vi "About.vi"() -> ()   [LabVIEW 2013]
panel:
  out "String":string="Advanced Plotting Toolkit Third-Party License Agreements And Acknowledgements\n========================================================\n\n\"This product includes color specifications and designs developed by\nCynthia Brewer (http://colorbrewer.org/).\"\n\n\nSilk Icons\n----------\n\nThis product makes use of the Silk Icon Set, released by Mark James under the\nCreative Commons Attribution 2.5 License.\n\nhttp://www.famfamfam.com/lab/icons/silk\n\n\nNumPy\n-----\n\nCopyright (c) 2005-2011, NumPy Developers.\nAll rights reserved.\n\nRedistribution and use in source and binary forms, with or without\nmodification, are permitted provided that the following conditions are\nmet:\n\n   Redistributions of source code must retain the above copyright\n       notice, this list of conditions and the following disclaimer.\n\n   Redistributions in binary form must reproduce the above\n       copyright notice, this list of conditions and the following\n       disclaimer in the documentation and/or other materials provided\n       with the distribution.\n\n   Neither the name of the NumPy Developers nor the names of any\n       contributors may be used to endorse or promote products derived\n       from this software without specific prior written permission.\n\nTHIS SOFTWARE IS PROVIDED BY THE COPYRIGHT HOLDERS AND CONTRIBUTORS\n\"AS IS\" AND ANY EXPRESS OR IMPLIED WARRANTIES, INCLUDING, BUT NOT\nLIMITED TO, THE IMPLIED WARRANTIES OF MERCHANTABILITY AND FITNESS FOR\nA PARTICULAR PURPOSE ARE DISCLAIMED. IN NO EVENT SHALL THE COPYRIGHT\nOWNER OR CONTRIBUTORS BE LIABLE FOR ANY DIRECT, INDIRECT, INCIDENTAL,\nSPECIAL, EXEMPLARY, OR CONSEQUENTIAL DAMAGES (INCLUDING, BUT NOT\nLIMITED TO, PROCUREMENT OF SUBSTITUTE GOODS OR SERVICES; LOSS OF USE,\nDATA, OR PROFITS; OR BUSINESS INTERRUPTION) HOWEVER CAUSED AND ON ANY\nTHEORY OF LIABILITY, WHETHER IN CONTRACT, STRICT LIABILITY, OR TORT\n(INCLUDING NEGLIGENCE OR OTHERWISE) ARISING IN ANY WAY OUT OF THE USE\nOF THIS SOFTWARE, EVEN IF ADVISED OF THE POSSIBILITY OF SUCH DAMAGE.\n\n\nNumPy (SafeEval)\n----------------\n\nCopyright 2006 Michael Spencer.  Released under the Python Software\nFoundation License (see \"Python 2.7\", below).\n\n\nNumPy (RandomKit)\n-----------------\n\nCopyright (c) 2003-2005, Jean-Sebastien Roy (js@jeannot.org)\n\nPermission is hereby granted, free of charge, to any person obtaining a\ncopy of this software and associated documentation files (the\n\"Software\"), to deal in the Software without restriction, including\nwithout limitation the rights to use, copy, modify, merge, publish,\ndistribute, sublicense, and/or sell copies of the Software, and to\npermit persons to whom the Software is furnished to do so, subject to\nthe following conditions:\n\nThe above copyright notice and this permission notice shall be included\nin all copies or substantial portions of the Software.\n\nTHE SOFTWARE IS PROVIDED \"AS IS\", WITHOUT WARRANTY OF ANY KIND, EXPRESS\nOR IMPLIED, INCLUDING BUT NOT LIMITED TO THE WARRANTIES OF\nMERCHANTABILITY, FITNESS FOR A PARTICULAR PURPOSE AND NONINFRINGEMENT.\nIN NO EVENT SHALL THE AUTHORS OR COPYRIGHT HOLDERS BE LIABLE FOR ANY\nCLAIM, DAMAGES OR OTHER LIABILITY, WHETHER IN AN ACTION OF CONTRACT,\nTORT OR OTHERWISE, ARISING FROM, OUT OF OR IN CONNECTION WITH THE\nSOFTWARE OR THE USE OR OTHER DEALINGS IN THE SOFTWARE.\n\n\nNumPy (rk_random, rk_seet, Mersenne Twister RNG)\n------------------------------------------------\n\nThe rk_random and rk_seed functions algorithms and the original design of\nthe Mersenne Twister RNG:\n\n  Copyright (C) 1997 - 2002, Makoto Matsumoto and Takuji Nishimura,\n  All rights reserved.\n\n  Redistribution and use in source and binary forms, with or without\n  modification, are permitted provided that the following conditions\n  are met:\n\n  1. Redistributions of source code must retain the above copyright\n  notice, this list of conditions and the following disclaimer.\n\n  2. Redistributions in binary form must reproduce the above copyright\n  notice, this list of conditions and the following disclaimer in the\n  documentation and/or other materials provided with the distribution.\n\n  3. The names of its contributors may not be used to endorse or promote\n  products derived from this software without specific prior written\n  permission.\n\n  THIS SOFTWARE IS PROVIDED BY THE COPYRIGHT HOLDERS AND CONTRIBUTORS\n  \"AS IS\" AND ANY EXPRESS OR IMPLIED WARRANTIES, INCLUDING, BUT NOT\n  LIMITED TO, THE IMPLIED WARRANTIES OF MERCHANTABILITY AND FITNESS FOR\n  A PARTICULAR PURPOSE ARE DISCLAIMED.  IN NO EVENT SHALL THE COPYRIGHT OWNER\n  OR CONTRIBUTORS BE LIABLE FOR ANY DIRECT, INDIRECT, INCIDENTAL, SPECIAL,\n  EXEMPLARY, OR CONSEQUENTIAL DAMAGES (INCLUDING, BUT NOT LIMITED TO,\n  PROCUREMENT OF SUBSTITUTE GOODS OR SERVICES; LOSS OF USE, DATA, OR\n  PROFITS; OR BUSINESS INTERRUPTION) HOWEVER CAUSED AND ON ANY THEORY OF\n  LIABILITY, WHETHER IN CONTRACT, STRICT LIABILITY, OR TORT (INCLUDING\n  NEGLIGENCE OR OTHERWISE) ARISING IN ANY WAY OUT OF THE USE OF THIS\n  SOFTWARE, EVEN IF ADVISED OF THE POSSIBILITY OF SUCH DAMAGE.\n  \n  \nNumPy (MSUN/npy_math)\n---------------------\n\nCopyright (C) 1993 by Sun Microsystems, Inc. All rights reserved.\n\nDeveloped at SunPro, a Sun Microsystems, Inc. business.\nPermission to use, copy, modify, and distribute this\nsoftware is freely granted, provided that this notice\nis preserved.\n\n\nNumPy (npy_math_complex)\n------------------------\n\nCopyright (c) 2007 David Schultz <das@FreeBSD.ORG>\nAll rights reserved.\n\nRedistribution and use in source and binary forms, with or without\nmodification, are permitted provided that the following conditions\nare met:\n1. Redistributions of source code must retain the above copyright\n   notice, this list of conditions and the following disclaimer.\n2. Redistributions in binary form must reproduce the above copyright\n   notice, this list of conditions and the following disclaimer in the\n   documentation and/or other materials provided with the distribution.\n\nTHIS SOFTWARE IS PROVIDED BY THE AUTHOR AND CONTRIBUTORS ``AS IS'' AND\nANY EXPRESS OR IMPLIED WARRANTIES, INCLUDING, BUT NOT LIMITED TO, THE\nIMPLIED WARRANTIES OF MERCHANTABILITY AND FITNESS FOR A PARTICULAR PURPOSE\nARE DISCLAIMED.  IN NO EVENT SHALL THE AUTHOR OR CONTRIBUTORS BE LIABLE\nFOR ANY DIRECT, INDIRECT, INCIDENTAL, SPECIAL, EXEMPLARY, OR CONSEQUENTIAL\nDAMAGES (INCLUDING, BUT NOT LIMITED TO, PROCUREMENT OF SUBSTITUTE GOODS\nOR SERVICES; LOSS OF USE, DATA, OR PROFITS; OR BUSINESS INTERRUPTION)\nHOWEVER CAUSED AND ON ANY THEORY OF LIABILITY, WHETHER IN CONTRACT, STRICT\nLIABILITY, OR TORT (INCLUDING NEGLIGENCE OR OTHERWISE) ARISING IN ANY WAY\nOUT OF THE USE OF THIS SOFTWARE, EVEN IF ADVISED OF THE POSSIBILITY OF\nSUCH DAMAGE.\n\n\nNumPy (mtrand)\n--------------\n\nCopyright 2005 Robert Kern (robert.kern@gmail.com)\n\nPermission is hereby granted, free of charge, to any person obtaining a\ncopy of this software and associated documentation files (the\n\"Software\"), to deal in the Software without restriction, including\nwithout limitation the rights to use, copy, modify, merge, publish,\ndistribute, sublicense, and/or sell copies of the Software, and to\npermit persons to whom the Software is furnished to do so, subject to\nthe following conditions:\n\nThe above copyright notice and this permission notice shall be included\nin all copies or substantial portions of the Software.\n\nTHE SOFTWARE IS PROVIDED \"AS IS\", WITHOUT WARRANTY OF ANY KIND, EXPRESS\nOR IMPLIED, INCLUDING BUT NOT LIMITED TO THE WARRANTIES OF\nMERCHANTABILITY, FITNESS FOR A PARTICULAR PURPOSE AND NONINFRINGEMENT.\nIN NO EVENT SHALL THE AUTHORS OR COPYRIGHT HOLDERS BE LIABLE FOR ANY\nCLAIM, DAMAGES OR OTHER LIABILITY, WHETHER IN AN ACTION OF CONTRACT,\nTORT OR OTHERWISE, ARISING FROM, OUT OF OR IN CONNECTION WITH THE\nSOFTWARE OR THE USE OR OTHER DEALINGS IN THE SOFTWARE.\n\n\nNumPy (fenv)\n------------\n\nCopyright (c) 2004 David Schultz <das@FreeBSD.ORG>\nAll rights reserved.\n\nRedistribution and use in source and binary forms, with or without\nmodification, are permitted provided that the following conditions\nare met:\n1. Redistributions of source code must retain the above copyright\n   notice, this list of conditions and the following disclaimer.\n2. Redistributions in binary form must reproduce the above copyright\n   notice, this list of conditions and the following disclaimer in the\n   documentation and/or other materials provided with the distribution.\n\nTHIS SOFTWARE IS PROVIDED BY THE AUTHOR AND CONTRIBUTORS ``AS IS'' AND\nANY EXPRESS OR IMPLIED WARRANTIES, INCLUDING, BUT NOT LIMITED TO, THE\nIMPLIED WARRANTIES OF MERCHANTABILITY AND FITNESS FOR A PARTICULAR PURPOSE\nARE DISCLAIMED.  IN NO EVENT SHALL THE AUTHOR OR CONTRIBUTORS BE LIABLE\nFOR ANY DIRECT, INDIRECT, INCIDENTAL, SPECIAL, EXEMPLARY, OR CONSEQUENTIAL\nDAMAGES (INCLUDING, BUT NOT LIMITED TO, PROCUREMENT OF SUBSTITUTE GOODS\nOR SERVICES; LOSS OF USE, DATA, OR PROFITS; OR BUSINESS INTERRUPTION)\nHOWEVER CAUSED AND ON ANY THEORY OF LIABILITY, WHETHER IN CONTRACT, STRICT\nLIABILITY, OR TORT (INCLUDING NEGLIGENCE OR OTHERWISE) ARISING IN ANY WAY\nOUT OF THE USE OF THIS SOFTWARE, EVEN IF ADVISED OF THE POSSIBILITY OF\nSUCH DAMAGE.\n\n\nMatplotlib\n----------\n\nLicense agreement for matplotlib 1.3.1 \n\n1. This LICENSE AGREEMENT is between the Matplotlib Development Team\n(“MDT”), and the Individual or Organization (“Licensee”) accessing and\notherwise using matplotlib software in source or binary form and its\nassociated documentation.\n\n2. Subject to the terms and conditions of this License Agreement, MDT\nhereby grants Licensee a nonexclusive, royalty-free, world-wide license\nto reproduce, analyze, test, perform and/or display publicly, prepare\nderivative works, distribute, and otherwise use matplotlib 1.3.1 alone\nor in any derivative version, provided, however, that MDT’s License\nAgreement and MDT’s notice of copyright, i.e., “Copyright (c) 2012-2013\nMatplotlib Development Team; All Rights Reserved” are retained in\nmatplotlib 1.3.1 alone or in any derivative version prepared by\nLicensee.\n\n3. In the event Licensee prepares a derivative work that is based on or\nincorporates matplotlib 1.3.1 or any part thereof, and wants to make the\nderivative work available to others as provided herein, then Licensee\nhereby agrees to include in any such work a brief summary of the changes\nmade to matplotlib 1.3.1.\n\n4. MDT is making matplotlib 1.3.1 available to Licensee on an “AS IS”\nbasis. MDT MAKES NO REPRESENTATIONS OR WARRANTIES, EXPRESS OR IMPLIED.\nBY WAY OF EXAMPLE, BUT NOT LIMITATION, MDT MAKES NO AND DISCLAIMS ANY\nREPRESENTATION OR WARRANTY OF MERCHANTABILITY OR FITNESS FOR ANY\nPARTICULAR PURPOSE OR THAT THE USE OF MATPLOTLIB 1.3.1 WILL NOT INFRINGE\nANY THIRD PARTY RIGHTS.\n\n5. MDT SHALL NOT BE LIABLE TO LICENSEE OR ANY OTHER USERS OF MATPLOTLIB\n1.3.1 FOR ANY INCIDENTAL, SPECIAL, OR CONSEQUENTIAL DAMAGES OR LOSS AS A\nRESULT OF MODIFYING, DISTRIBUTING, OR OTHERWISE USING MATPLOTLIB 1.3.1,\nOR ANY DERIVATIVE THEREOF, EVEN IF ADVISED OF THE POSSIBILITY THEREOF.\n\n6. This License Agreement will automatically terminate upon a material\nbreach of its terms and conditions.\n\n7. Nothing in this License Agreement shall be deemed to create any\nrelationship of agency, partnership, or joint venture between MDT and\nLicensee. This License Agreement does not grant permission to use MDT\ntrademarks or trade name in a trademark sense to endorse or promote\nproducts or services of Licensee, or any third party.\n\n8. By copying, installing or otherwise using matplotlib 1.3.1, Licensee\nagrees to be bound by the terms and conditions of this License Agreement.\n\n\nMatplotlib (PyCXX)\n------------------\n\nCopyright (c) 1998 - 2007, The Regents of the University of California\nProduced at the Lawrence Livermore National Laboratory\nAll rights reserved.\n\nThis file is part of PyCXX. For details,see http:cxx.sourceforge.net/. The\nfull copyright notice is contained in the file COPYRIGHT located at the root\nof the PyCXX distribution.\n\nRedistribution  and  use  in  source  and  binary  forms,  with  or  without\nmodification, are permitted provided that the following conditions are met:\n\n - Redistributions of  source code must  retain the above  copyright notice,\n   this list of conditions and the disclaimer below.\n - Redistributions in binary form must reproduce the above copyright notice,\n   this  list of  conditions  and  the  disclaimer (as noted below)  in  the\n   documentation and/or materials provided with the distribution.\n - Neither the name of the UC/LLNL nor  the names of its contributors may be\n   used to  endorse or  promote products derived from  this software without\n   specific prior written permission.\n\nTHIS SOFTWARE IS PROVIDED BY THE COPYRIGHT  HOLDERS AND CONTRIBUTORS \"AS IS\"\nAND ANY EXPRESS OR  IMPLIED WARRANTIES, INCLUDING,  BUT NOT  LIMITED TO, THE\nIMPLIED WARRANTIES OF MERCHANTABILITY AND  FITNESS FOR A PARTICULAR  PURPOSE\nARE  DISCLAIMED.  IN  NO  EVENT  SHALL  THE  REGENTS  OF  THE  UNIVERSITY OF\nCALIFORNIA, THE U.S.  DEPARTMENT  OF  ENERGY OR CONTRIBUTORS BE  LIABLE  FOR\nANY  DIRECT,  INDIRECT,  INCIDENTAL,  SPECIAL,  EXEMPLARY,  OR CONSEQUENTIAL\nDAMAGES (INCLUDING, BUT NOT  LIMITED TO, PROCUREMENT OF  SUBSTITUTE GOODS OR\nSERVICES; LOSS OF  USE, DATA, OR PROFITS; OR  BUSINESS INTERRUPTION) HOWEVER\nCAUSED  AND  ON  ANY  THEORY  OF  LIABILITY,  WHETHER  IN  CONTRACT,  STRICT\nLIABILITY, OR TORT  (INCLUDING NEGLIGENCE OR OTHERWISE)  ARISING IN ANY  WAY\nOUT OF THE  USE OF THIS SOFTWARE, EVEN IF ADVISED OF THE POSSIBILITY OF SUCH\nDAMAGE.\n\n\nMatplotlib (Agg)\n----------------\n\nThe Anti-Grain Geometry Project\nA high quality rendering engine for C++\nhttp://antigrain.com\n\nAnti-Grain Geometry - Version 2.4 \nCopyright (C) 2002-2005 Maxim Shemanarev (McSeem) \n\nPermission to copy, use, modify, sell and distribute this software \nis granted provided this copyright notice appears in all copies. \nThis software is provided \"as is\" without express or implied\nwarranty, and with no claim as to its suitability for any purpose.\n\n\nMatplotlib (VoronoiDiagram)\n---------------------------\n\nThe author of this software is Steven Fortune.  Copyright (c) 1994 by AT&T\nBell Laboratories.\n\nPermission to use, copy, modify, and distribute this software for any\npurpose without fee is hereby granted, provided that this entire notice\nis included in all copies of any software which is or includes a copy\nor modification of this software and in all copies of the supporting\ndocumentation for such software.\n\nTHIS SOFTWARE IS BEING PROVIDED \"AS IS\", WITHOUT ANY EXPRESS OR IMPLIED\nWARRANTY.  IN PARTICULAR, NEITHER THE AUTHORS NOR AT&T MAKE ANY\nREPRESENTATION OR WARRANTY OF ANY KIND CONCERNING THE MERCHANTABILITY\nOF THIS SOFTWARE OR ITS FITNESS FOR ANY PARTICULAR PURPOSE.\n\n\nMatplotlib (Delauney Triangulation)\n-----------------------------------\n\n(c) Robert Kern, under the SciPy License (follows)\n\nCopyright (c) 2001, 2002 Enthought, Inc.\nAll rights reserved.\n\nCopyright (c) 2003-2013 SciPy Developers.\n\nRedistribution and use in source and binary forms, with or without\nmodification, are permitted provided that the following conditions are\nmet:\n\nRedistributions of source code must retain the above copyright notice,\nthis list of conditions and the following disclaimer. Redistributions in\nbinary form must reproduce the above copyright notice, this list of\nconditions and the following disclaimer in the documentation and/or\nother materials provided with the distribution. Neither the name of\nEnthought nor the names of the SciPy Developers may be used to endorse\nor promote products derived from this software without specific prior\nwritten permission. \n\nTHIS SOFTWARE IS PROVIDED BY THE COPYRIGHT HOLDERS\nAND CONTRIBUTORS “AS IS” AND ANY EXPRESS OR IMPLIED WARRANTIES,\nINCLUDING, BUT NOT LIMITED TO, THE IMPLIED WARRANTIES OF MERCHANTABILITY\nAND FITNESS FOR A PARTICULAR PURPOSE ARE DISCLAIMED. IN NO EVENT SHALL\nTHE REGENTS OR CONTRIBUTORS BE LIABLE FOR ANY DIRECT, INDIRECT,\nINCIDENTAL, SPECIAL, EXEMPLARY, OR CONSEQUENTIAL DAMAGES (INCLUDING, BUT\nNOT LIMITED TO, PROCUREMENT OF SUBSTITUTE GOODS OR SERVICES; LOSS OF\nUSE, DATA, OR PROFITS; OR BUSINESS INTERRUPTION) HOWEVER CAUSED AND ON\nANY THEORY OF LIABILITY, WHETHER IN CONTRACT, STRICT LIABILITY, OR TORT\n(INCLUDING NEGLIGENCE OR OTHERWISE) ARISING IN ANY WAY OUT OF THE USE OF\nTHIS SOFTWARE, EVEN IF ADVISED OF THE POSSIBILITY OF SUCH DAMAGE.\n\n\nMatplotlib (BaKoMa Fonts)\n-------------------------\n\nBaKoMa Fonts Licence\n\n  This licence covers two font packs (known as BaKoMa Fonts Colelction,\n  which is available at `CTAN:fonts/cm/ps-type1/bakoma/'):\n\n    1) BaKoMa-CM (1.1/12-Nov-94)\n       Computer Modern Fonts in PostScript Type 1 and TrueType font formats.\n\n    2) BaKoMa-AMS (1.2/19-Jan-95)\n       AMS TeX fonts in PostScript Type 1 and TrueType font formats.\n   \n  Copyright (C) 1994, 1995, Basil K. Malyshev. All Rights Reserved.\n\n  Permission to copy and distribute these fonts for any purpose is \n  hereby granted without fee, provided that the above copyright notice, \n  author statement and this permission notice appear in all copies of \n  these fonts and related documentation.\n\n  Permission to modify and distribute modified fonts for any purpose is \n  hereby granted without fee, provided that the copyright notice, \n  author statement, this permission notice and location of original \n  fonts (http://www.ctan.org/tex-archive/fonts/cm/ps-type1/bakoma)\n  appear in all copies of modified fonts and related documentation.\n\n  Permission to use these fonts (embedding into PostScript, PDF, SVG\n  and printing by using any software) is hereby granted without fee. \n  It is not required to provide any notices about using these fonts.\n\n Basil K. Malyshev\n INSTITUTE FOR HIGH ENERGY PHYSICS\n IHEP, OMVT\n Moscow Region\n 142281 PROTVINO\n RUSSIA\n\n E-Mail:\tbakoma@mail.ru\n      or\tmalyshev@mail.ihep.ru\n      \n      \nMatplotlib (ColorBrewer)\n------------------------\n\nApache-Style Software License for ColorBrewer Color Schemes\n\nVersion 1.1\n\nCopyright (c) 2002 Cynthia Brewer, Mark Harrower, and The Pennsylvania \nState University. All rights reserved. Redistribution and use in source \nand binary forms, with or without modification, are permitted provided \nthat the following conditions are met:\n\n1. Redistributions as source code must retain the above copyright notice, \nthis list of conditions and the following disclaimer.\n\n2. The end-user documentation included with the redistribution, if any, \nmust include the following acknowledgment: \"This product includes color \nspecifications and designs developed by Cynthia Brewer \n(http://colorbrewer.org/).\" Alternately, this acknowledgment may appear in \nthe software itself, if and wherever such third-party acknowledgments \nnormally appear.\n\n3. The name \"ColorBrewer\" must not be used to endorse or promote products \nderived from this software without prior written permission. For written \npermission, please contact Cynthia Brewer at cbrewer@psu.edu.\n\n4. Products derived from this software may not be called \"ColorBrewer\", \nnor may \"ColorBrewer\" appear in their name, without prior written \npermission of Cynthia Brewer.\n\nTHIS SOFTWARE IS PROVIDED \"AS IS\" AND ANY EXPRESSED OR IMPLIED WARRANTIES, \nINCLUDING, BUT NOT LIMITED TO, THE IMPLIED WARRANTIES OF MERCHANTABILITY \nAND FITNESS FOR A PARTICULAR PURPOSE ARE DISCLAIMED. IN NO EVENT SHALL \nCYNTHIA BREWER, MARK HARROWER, OR THE PENNSYLVANIA STATE UNIVERSITY BE \nLIABLE FOR ANY DIRECT, INDIRECT, INCIDENTAL, SPECIAL, EXEMPLARY, OR \nCONSEQUENTIAL DAMAGES (INCLUDING, BUT NOT LIMITED TO, PROCUREMENT OF \nSUBSTITUTE GOODS OR SERVICES; LOSS OF USE, DATA, OR PROFITS; OR BUSINESS \nINTERRUPTION) HOWEVER CAUSED AND ON ANY THEORY OF LIABILITY, WHETHER IN \nCONTRACT, STRICT LIABILITY, OR TORT (INCLUDING NEGLIGENCE OR OTHERWISE) \nARISING IN ANY WAY OUT OF THE USE OF THIS SOFTWARE, EVEN IF ADVISED OF THE \nPOSSIBILITY OF SUCH DAMAGE.\n\n\nMatplotlib (Enthought Contributions)\n------------------------------------\n\nCopyright (c) 2001, 2002 Enthought, Inc.\n\nAll rights reserved.\n\nRedistribution and use in source and binary forms, with or without\nmodification, are permitted provided that the following conditions are met:\n\n  a. Redistributions of source code must retain the above copyright notice,\n     this list of conditions and the following disclaimer.\n  b. Redistributions in binary form must reproduce the above copyright\n     notice, this list of conditions and the following disclaimer in the\n     documentation and/or other materials provided with the distribution.\n  c. Neither the name of the Enthought nor the names of its contributors\n     may be used to endorse or promote products derived from this software\n     without specific prior written permission.\n\n\nTHIS SOFTWARE IS PROVIDED BY THE COPYRIGHT HOLDERS AND CONTRIBUTORS \"AS IS\"\nAND ANY EXPRESS OR IMPLIED WARRANTIES, INCLUDING, BUT NOT LIMITED TO, THE\nIMPLIED WARRANTIES OF MERCHANTABILITY AND FITNESS FOR A PARTICULAR PURPOSE\nARE DISCLAIMED. IN NO EVENT SHALL THE REGENTS OR CONTRIBUTORS BE LIABLE FOR\nANY DIRECT, INDIRECT, INCIDENTAL, SPECIAL, EXEMPLARY, OR CONSEQUENTIAL\nDAMAGES (INCLUDING, BUT NOT LIMITED TO, PROCUREMENT OF SUBSTITUTE GOODS OR\nSERVICES; LOSS OF USE, DATA, OR PROFITS; OR BUSINESS INTERRUPTION) HOWEVER\nCAUSED AND ON ANY THEORY OF LIABILITY, WHETHER IN CONTRACT, STRICT\nLIABILITY, OR TORT (INCLUDING NEGLIGENCE OR OTHERWISE) ARISING IN ANY WAY\nOUT OF THE USE OF THIS SOFTWARE, EVEN IF ADVISED OF THE POSSIBILITY OF SUCH\nDAMAGE.\n\n\nMatplotlib (Formlayout)\n-----------------------\n\nCopyright (c) 2009 Pierre Raybaut\n\nPermission is hereby granted, free of charge, to any person\nobtaining a copy of this software and associated documentation\nfiles (the \"Software\"), to deal in the Software without\nrestriction, including without limitation the rights to use,\ncopy, modify, merge, publish, distribute, sublicense, and/or sell\ncopies of the Software, and to permit persons to whom the\nSoftware is furnished to do so, subject to the following\nconditions:\n\nThe above copyright notice and this permission notice shall be\nincluded in all copies or substantial portions of the Software.\n\nTHE SOFTWARE IS PROVIDED \"AS IS\", WITHOUT WARRANTY OF ANY KIND,\nEXPRESS OR IMPLIED, INCLUDING BUT NOT LIMITED TO THE WARRANTIES\nOF MERCHANTABILITY, FITNESS FOR A PARTICULAR PURPOSE AND\nNONINFRINGEMENT. IN NO EVENT SHALL THE AUTHORS OR COPYRIGHT\nHOLDERS BE LIABLE FOR ANY CLAIM, DAMAGES OR OTHER LIABILITY,\nWHETHER IN AN ACTION OF CONTRACT, TORT OR OTHERWISE, ARISING\nFROM, OUT OF OR IN CONNECTION WITH THE SOFTWARE OR THE USE OR\nOTHER DEALINGS IN THE SOFTWARE.\n\n\nMatplotlib (STIX Fonts)\n-----------------------\n\nCopyright (c) 2001-2010 by the STI Pub Companies, consisting of the American\nInstitute of Physics, the American Chemical Society, the American Mathematical\nSociety, the American Physical Society, Elsevier, Inc., and The Institute of\nElectrical and Electronic Engineers, Inc. (www.stixfonts.org), with Reserved\nFont Name STIX Fonts, STIX Fonts (TM) is a  trademark of The Institute of\nElectrical and Electronics Engineers, Inc.\n\nPortions copyright (c) 1998-2003 by MicroPress, Inc. (www.micropress-inc.com),\nwith Reserved Font Name TM Math. To obtain additional mathematical fonts, please\ncontact MicroPress, Inc., 68-30 Harrow Street, Forest Hills, NY 11375, USA,\nPhone: (718) 575-1816.\n\nPortions copyright (c) 1990 by Elsevier, Inc.\n\nThis Font Software is licensed under the SIL Open Font License, Version 1.1.\nThis license is copied below, and is also available with a FAQ at:\nhttp://scripts.sil.org/OFL\n\n-----------------------------------------------------------\nSIL OPEN FONT LICENSE Version 1.1 - 26 February 2007\n-----------------------------------------------------------\n\nPREAMBLE\nThe goals of the Open Font License (OFL) are to stimulate worldwide\ndevelopment of collaborative font projects, to support the font creation\nefforts of academic and linguistic communities, and to provide a free and\nopen framework in which fonts may be shared and improved in partnership\nwith others.\n\nThe OFL allows the licensed fonts to be used, studied, modified and\nredistributed freely as long as they are not sold by themselves. The\nfonts, including any derivative works, can be bundled, embedded,\nredistributed and/or sold with any software provided that any reserved\nnames are not used by derivative works. The fonts and derivatives,\nhowever, cannot be released under any other type of license. The\nrequirement for fonts to remain under this license does not apply\nto any document created using the fonts or their derivatives.\n\nDEFINITIONS\n\"Font Software\" refers to the set of files released by the Copyright\nHolder(s) under this license and clearly marked as such. This may\ninclude source files, build scripts and documentation.\n\n\"Reserved Font Name\" refers to any names specified as such after the\ncopyright statement(s).\n\n\"Original Version\" refers to the collection of Font Software components as\ndistributed by the Copyright Holder(s).\n\n\"Modified Version\" refers to any derivative made by adding to, deleting,\nor substituting -- in part or in whole -- any of the components of the\nOriginal Version, by changing formats or by porting the Font Software to a\nnew environment.\n\n\"Author\" refers to any designer, engineer, programmer, technical\nwriter or other person who contributed to the Font Software.\n\nPERMISSION & CONDITIONS\nPermission is hereby granted, free of charge, to any person obtaining\na copy of the Font Software, to use, study, copy, merge, embed, modify,\nredistribute, and sell modified and unmodified copies of the Font\nSoftware, subject to the following conditions:\n\n1) Neither the Font Software nor any of its individual components,\nin Original or Modified Versions, may be sold by itself.\n\n2) Original or Modified Versions of the Font Software may be bundled,\nredistributed and/or sold with any software, provided that each copy\ncontains the above copyright notice and this license. These can be\nincluded either as stand-alone text files, human-readable headers or\nin the appropriate machine-readable metadata fields within text or\nbinary files as long as those fields can be easily viewed by the user.\n\n3) No Modified Version of the Font Software may use the Reserved Font\nName(s) unless explicit written permission is granted by the corresponding\nCopyright Holder. This restriction only applies to the primary font name as\npresented to the users.\n\n4) The name(s) of the Copyright Holder(s) or the Author(s) of the Font\nSoftware shall not be used to promote, endorse or advertise any\nModified Version, except to acknowledge the contribution(s) of the\nCopyright Holder(s) and the Author(s) or with their explicit written\npermission.\n\n5) The Font Software, modified or unmodified, in part or in whole,\nmust be distributed entirely under this license, and must not be\ndistributed under any other license. The requirement for fonts to\nremain under this license does not apply to any document created\nusing the Font Software.\n\nTERMINATION\nThis license becomes null and void if any of the above conditions are\nnot met.\n\nDISCLAIMER\nTHE FONT SOFTWARE IS PROVIDED \"AS IS\", WITHOUT WARRANTY OF ANY KIND,\nEXPRESS OR IMPLIED, INCLUDING BUT NOT LIMITED TO ANY WARRANTIES OF\nMERCHANTABILITY, FITNESS FOR A PARTICULAR PURPOSE AND NONINFRINGEMENT\nOF COPYRIGHT, PATENT, TRADEMARK, OR OTHER RIGHT. IN NO EVENT SHALL THE\nCOPYRIGHT HOLDER BE LIABLE FOR ANY CLAIM, DAMAGES OR OTHER LIABILITY,\nINCLUDING ANY GENERAL, SPECIAL, INDIRECT, INCIDENTAL, OR CONSEQUENTIAL\nDAMAGES, WHETHER IN AN ACTION OF CONTRACT, TORT OR OTHERWISE, ARISING\nFROM, OUT OF THE USE OR INABILITY TO USE THE FONT SOFTWARE OR FROM\nOTHER DEALINGS IN THE FONT SOFTWARE.\n\n\nMatplotlib (GIST/Yorick Colormaps)\n----------------------------------\n\n  Copyright (c) 1996.  The Regents of the University of California.\n\t\t\t All rights reserved.\n\nPermission to use, copy, modify, and distribute this software for any\npurpose without fee is hereby granted, provided that this entire\nnotice is included in all copies of any software which is or includes\na copy or modification of this software and in all copies of the\nsupporting documentation for such software.\n\nThis work was produced at the University of California, Lawrence\nLivermore National Laboratory under contract no. W-7405-ENG-48 between\nthe U.S. Department of Energy and The Regents of the University of\nCalifornia for the operation of UC LLNL.\n\n\n\t\t\t      DISCLAIMER\n\nThis software was prepared as an account of work sponsored by an\nagency of the United States Government.  Neither the United States\nGovernment nor the University of California nor any of their\nemployees, makes any warranty, express or implied, or assumes any\nliability or responsibility for the accuracy, completeness, or\nusefulness of any information, apparatus, product, or process\ndisclosed, or represents that its use would not infringe\nprivately-owned rights.  Reference herein to any specific commercial\nproducts, process, or service by trade name, trademark, manufacturer,\nor otherwise, does not necessarily constitute or imply its\nendorsement, recommendation, or favoring by the United States\nGovernment or the University of California.  The views and opinions of\nauthors expressed herein do not necessarily state or reflect those of\nthe United States Government or the University of California, and\nshall not be used for advertising or product endorsement purposes.\n\n\n\t\t\t\tAUTHOR\n\nDavid H. Munro wrote Yorick and Gist.  Berkeley Yacc (byacc) generated\nthe Yorick parser.  The routines in Math are from LAPACK and FFTPACK;\nMathC contains C translations by David H. Munro.  The algorithms for\nYorick's random number generator and several special functions in\nYorick/include were taken from Numerical Recipes by Press, et. al.,\nalthough the Yorick implementations are unrelated to those in\nNumerical Recipes.  A small amount of code in Gist was adapted from\nthe X11R4 release, copyright M.I.T. -- the complete copyright notice\nmay be found in the (unused) file Gist/host.c.\n\n\nMatplotlib (Pnpoly)\n-------------------\n\nCopyright (c) 1970-2003, Wm. Randolph Franklin\n\nPermission is hereby granted, free of charge, to any person obtaining\na copy of this software and associated documentation files (the\n\"Software\"), to deal in the Software without restriction, including\nwithout limitation the rights to use, copy, modify, merge, publish,\ndistribute, sublicense, and/or sell copies of the Software, and to\npermit persons to whom the Software is furnished to do so, subject to\nthe following conditions:\n\n   1. Redistributions of source code must retain the above copyright\n      notice, this list of conditions and the following disclaimers.\n   2. Redistributions in binary form must reproduce the above\n      copyright notice in the documentation and/or other materials\n      provided with the distribution.\n   3. The name of W. Randolph Franklin may not be used to endorse or\n      promote products derived from this Software without specific\n      prior written permission. \n\nTHE SOFTWARE IS PROVIDED \"AS IS\", WITHOUT WARRANTY OF ANY KIND,\nEXPRESS OR IMPLIED, INCLUDING BUT NOT LIMITED TO THE WARRANTIES OF\nMERCHANTABILITY, FITNESS FOR A PARTICULAR PURPOSE AND\nNONINFRINGEMENT. IN NO EVENT SHALL THE AUTHORS OR COPYRIGHT HOLDERS BE\nLIABLE FOR ANY CLAIM, DAMAGES OR OTHER LIABILITY, WHETHER IN AN ACTION\nOF CONTRACT, TORT OR OTHERWISE, ARISING FROM, OUT OF OR IN CONNECTION\nWITH THE SOFTWARE OR THE USE OR OTHER DEALINGS IN THE SOFTWARE.\n\n\nMatplotlib (ttconv)\n-------------------\n\nCopyright 1995, Trinity College Computing Center.\nWritten by David Chappell.\n\nPermission to use, copy, modify, and distribute this software and its\ndocumentation for any purpose and without fee is hereby granted, provided\nthat the above copyright notice appear in all copies and that both that\ncopyright notice and this permission notice appear in supporting\ndocumentation.  This software is provided \"as is\" without express or\nimplied warranty.\n\n\nMatplotlib (Bitstream Vera)\n---------------------------\n\nBitstream Vera Fonts Copyright\n\nThe fonts have a generous copyright, allowing derivative works (as\nlong as \"Bitstream\" or \"Vera\" are not in the names), and full\nredistribution (so long as they are not sold by themselves). They\ncan be be bundled, redistributed and sold with any software.\n\nThe fonts are distributed under the following copyright:\n\nCopyright (c) 2003 by Bitstream, Inc. All Rights Reserved. Bitstream\nVera is a trademark of Bitstream, Inc.\n\nPermission is hereby granted, free of charge, to any person obtaining\na copy of the fonts accompanying this license (\"Fonts\") and associated\ndocumentation files (the \"Font Software\"), to reproduce and distribute\nthe Font Software, including without limitation the rights to use,\ncopy, merge, publish, distribute, and/or sell copies of the Font\nSoftware, and to permit persons to whom the Font Software is furnished\nto do so, subject to the following conditions:\n\nThe above copyright and trademark notices and this permission notice\nshall be included in all copies of one or more of the Font Software\ntypefaces.\n\nThe Font Software may be modified, altered, or added to, and in\nparticular the designs of glyphs or characters in the Fonts may be\nmodified and additional glyphs or characters may be added to the\nFonts, only if the fonts are renamed to names not containing either\nthe words \"Bitstream\" or the word \"Vera\".\n\nThis License becomes null and void to the extent applicable to Fonts\nor Font Software that has been modified and is distributed under the\n\"Bitstream Vera\" names.\n\nThe Font Software may be sold as part of a larger software package but\nno copy of one or more of the Font Software typefaces may be sold by\nitself.\n\nTHE FONT SOFTWARE IS PROVIDED \"AS IS\", WITHOUT WARRANTY OF ANY KIND,\nEXPRESS OR IMPLIED, INCLUDING BUT NOT LIMITED TO ANY WARRANTIES OF\nMERCHANTABILITY, FITNESS FOR A PARTICULAR PURPOSE AND NONINFRINGEMENT\nOF COPYRIGHT, PATENT, TRADEMARK, OR OTHER RIGHT. IN NO EVENT SHALL\nBITSTREAM OR THE GNOME FOUNDATION BE LIABLE FOR ANY CLAIM, DAMAGES OR\nOTHER LIABILITY, INCLUDING ANY GENERAL, SPECIAL, INDIRECT, INCIDENTAL,\nOR CONSEQUENTIAL DAMAGES, WHETHER IN AN ACTION OF CONTRACT, TORT OR\nOTHERWISE, ARISING FROM, OUT OF THE USE OR INABILITY TO USE THE FONT\nSOFTWARE OR FROM OTHER DEALINGS IN THE FONT SOFTWARE.\n\nExcept as contained in this notice, the names of Gnome, the Gnome\nFoundation, and Bitstream Inc., shall not be used in advertising or\notherwise to promote the sale, use or other dealings in this Font\nSoftware without prior written authorization from the Gnome Foundation\nor Bitstream Inc., respectively. For further information, contact:\nfonts at gnome dot org.\n\n\nMatplotlib (14 PDF Core Fonts)\n------------------------------\n\nFont Metrics for the 14 PDF Core Fonts (README from the Matplotlib\npackage):\n\nThis directory contains font metrics for the 14 PDF Core Fonts,\ndownloaded from Adobe. The title and this paragraph were added by\nMatplotlib developers. The download URL was\n<http://partners.adobe.com/public/developer/font/index.html>.\n\nThis file and the 14 PostScript(R) AFM files it accompanies may be used,\ncopied, and distributed for any purpose and without charge, with or\nwithout modification, provided that all copyright notices are retained;\nthat the AFM files are not distributed without this file; that all\nmodifications to this file or any of the AFM files are prominently noted\nin the modified file(s); and that this paragraph is not modified. Adobe\nSystems has no responsibility or obligation to support the use of the\nAFM files.\n\n\nMatplotlib (IPython Numutils)\n-----------------------------\n\nCopyright (c) 2001-2004, Fernando Perez. <Fernando.Perez@colorado.edu>\nAll rights reserved.\n\nThis license was generated from the BSD license template as found in:\nhttp://www.opensource.org/licenses/bsd-license.php\n\nRedistribution and use in source and binary forms, with or without\nmodification, are permitted provided that the following conditions are met:\n\n    Redistributions of source code must retain the above copyright notice,\n      this list of conditions and the following disclaimer.\n\n    Redistributions in binary form must reproduce the above copyright\n      notice, this list of conditions and the following disclaimer in the\n      documentation and/or other materials provided with the distribution.\n\n    Neither the name of the IPython project nor the names of its\n      contributors may be used to endorse or promote products derived from\n      this software without specific prior written permission.\n\nTHIS SOFTWARE IS PROVIDED BY THE COPYRIGHT HOLDERS AND CONTRIBUTORS \"AS IS\"\nAND ANY EXPRESS OR IMPLIED WARRANTIES, INCLUDING, BUT NOT LIMITED TO, THE\nIMPLIED WARRANTIES OF MERCHANTABILITY AND FITNESS FOR A PARTICULAR PURPOSE ARE\nDISCLAIMED. IN NO EVENT SHALL THE COPYRIGHT OWNER OR CONTRIBUTORS BE LIABLE\nFOR ANY DIRECT, INDIRECT, INCIDENTAL, SPECIAL, EXEMPLARY, OR CONSEQUENTIAL\nDAMAGES (INCLUDING, BUT NOT LIMITED TO, PROCUREMENT OF SUBSTITUTE GOODS OR\nSERVICES; LOSS OF USE, DATA, OR PROFITS; OR BUSINESS INTERRUPTION) HOWEVER\nCAUSED AND ON ANY THEORY OF LIABILITY, WHETHER IN CONTRACT, STRICT LIABILITY,\nOR TORT (INCLUDING NEGLIGENCE OR OTHERWISE) ARISING IN ANY WAY OUT OF THE USE\nOF THIS SOFTWARE, EVEN IF ADVISED OF THE POSSIBILITY OF SUCH DAMAGE.\n\n\nPython 2.7\n----------\n\nPYTHON SOFTWARE FOUNDATION LICENSE VERSION 2\n--------------------------------------------\n\n1. This LICENSE AGREEMENT is between the Python Software Foundation\n(\"PSF\"), and the Individual or Organization (\"Licensee\") accessing and\notherwise using this software (\"Python\") in source or binary form and\nits associated documentation.\n\n2. Subject to the terms and conditions of this License Agreement, PSF\nhereby grants Licensee a nonexclusive, royalty-free, world-wide\nlicense to reproduce, analyze, test, perform and/or display publicly,\nprepare derivative works, distribute, and otherwise use Python\nalone or in any derivative version, provided, however, that PSF's\nLicense Agreement and PSF's notice of copyright, i.e., \"Copyright (c)\n2001, 2002, 2003, 2004, 2005, 2006 Python Software Foundation; All Rights\nReserved\" are retained in Python alone or in any derivative version \nprepared by Licensee.\n\n3. In the event Licensee prepares a derivative work that is based on\nor incorporates Python or any part thereof, and wants to make\nthe derivative work available to others as provided herein, then\nLicensee hereby agrees to include in any such work a brief summary of\nthe changes made to Python.\n\n4. PSF is making Python available to Licensee on an \"AS IS\"\nbasis.  PSF MAKES NO REPRESENTATIONS OR WARRANTIES, EXPRESS OR\nIMPLIED.  BY WAY OF EXAMPLE, BUT NOT LIMITATION, PSF MAKES NO AND\nDISCLAIMS ANY REPRESENTATION OR WARRANTY OF MERCHANTABILITY OR FITNESS\nFOR ANY PARTICULAR PURPOSE OR THAT THE USE OF PYTHON WILL NOT\nINFRINGE ANY THIRD PARTY RIGHTS.\n\n5. PSF SHALL NOT BE LIABLE TO LICENSEE OR ANY OTHER USERS OF PYTHON\nFOR ANY INCIDENTAL, SPECIAL, OR CONSEQUENTIAL DAMAGES OR LOSS AS\nA RESULT OF MODIFYING, DISTRIBUTING, OR OTHERWISE USING PYTHON,\nOR ANY DERIVATIVE THEREOF, EVEN IF ADVISED OF THE POSSIBILITY THEREOF.\n\n6. This License Agreement will automatically terminate upon a material\nbreach of its terms and conditions.\n\n7. Nothing in this License Agreement shall be deemed to create any\nrelationship of agency, partnership, or joint venture between PSF and\nLicensee.  This License Agreement does not grant permission to use PSF\ntrademarks or trade name in a trademark sense to endorse or promote\nproducts or services of Licensee, or any third party.\n\n8. By copying, installing or otherwise using Python, Licensee\nagrees to be bound by the terms and conditions of this License\nAgreement.\n\n\nPyWin32\n-------\n\nCopyright (c) 1996-2008, Greg Stein and Mark Hammond.\nAll rights reserved.\n\nRedistribution and use in source and binary forms, with or without \nmodification, are permitted provided that the following conditions \nare met:\n\nRedistributions of source code must retain the above copyright notice, \nthis list of conditions and the following disclaimer.\n\nRedistributions in binary form must reproduce the above copyright \nnotice, this list of conditions and the following disclaimer in \nthe documentation and/or other materials provided with the distribution.\n\nNeither names of Greg Stein, Mark Hammond nor the name of contributors may be used \nto endorse or promote products derived from this software without \nspecific prior written permission. \n\nTHIS SOFTWARE IS PROVIDED BY THE COPYRIGHT HOLDERS AND CONTRIBUTORS ``AS\nIS'' AND ANY EXPRESS OR IMPLIED WARRANTIES, INCLUDING, BUT NOT LIMITED\nTO, THE IMPLIED WARRANTIES OF MERCHANTABILITY AND FITNESS FOR A\nPARTICULAR PURPOSE ARE DISCLAIMED. IN NO EVENT SHALL THE REGENTS OR\nCONTRIBUTORS BE LIABLE FOR ANY DIRECT, INDIRECT, INCIDENTAL, SPECIAL,\nEXEMPLARY, OR CONSEQUENTIAL DAMAGES (INCLUDING, BUT NOT LIMITED TO,\nPROCUREMENT OF SUBSTITUTE GOODS OR SERVICES; LOSS OF USE, DATA, OR\nPROFITS; OR BUSINESS INTERRUPTION) HOWEVER CAUSED AND ON ANY THEORY OF\nLIABILITY, WHETHER IN CONTRACT, STRICT LIABILITY, OR TORT (INCLUDING\nNEGLIGENCE OR OTHERWISE) ARISING IN ANY WAY OUT OF THE USE OF THIS\nSOFTWARE, EVEN IF ADVISED OF THE POSSIBILITY OF SUCH DAMAGE.\n\n\nPyWin32 (Scintilla portions)\n----------------------------\n\nCopyright 1998-2003 by Neil Hodgson <neilh@scintilla.org>\n\nAll Rights Reserved \n\nPermission to use, copy, modify, and distribute this software and its \ndocumentation for any purpose and without fee is hereby granted, \nprovided that the above copyright notice appear in all copies and that \nboth that copyright notice and this permission notice appear in \nsupporting documentation. \n\nNEIL HODGSON DISCLAIMS ALL WARRANTIES WITH REGARD TO THIS \nSOFTWARE, INCLUDING ALL IMPLIED WARRANTIES OF MERCHANTABILITY \nAND FITNESS, IN NO EVENT SHALL NEIL HODGSON BE LIABLE FOR ANY \nSPECIAL, INDIRECT OR CONSEQUENTIAL DAMAGES OR ANY DAMAGES \nWHATSOEVER RESULTING FROM LOSS OF USE, DATA OR PROFITS, \nWHETHER IN AN ACTION OF CONTRACT, NEGLIGENCE OR OTHER \nTORTIOUS ACTION, ARISING OUT OF OR IN CONNECTION WITH THE USE \nOR PERFORMANCE OF THIS SOFTWARE.\n\n\nPyWin32 (win32wnet)\n-------------------\n\nCopyright (c) 1998-1999 Cisco Systems, Inc. All Rights Reserved\nPermission to use, copy, modify, and distribute this software and its\ndocumentation for any purpose and without fee is hereby granted,\nprovided that the above copyright notice appear in all copies and that\nboth that copyright notice and this permission notice appear in\nsupporting documentation.\n\nCISCO SYSTEMS, INC. DISCLAIMS ALL WARRANTIES WITH REGARD TO THIS\nSOFTWARE, INCLUDING ALL IMPLIED WARRANTIES OF MERCHANTABILITY AND\nFITNESS. IN NO EVENT SHALL CISCO SYSTEMS BE LIABLE FOR ANY LOST REVENUE, \nPROFIT OR DATA, OR FOR SPECIAL, INDIRECT, CONSEQUENTIAL OR INCIDENTAL\nDAMAGES OR ANY OTHER DAMAGES WHATSOEVER, HOWEVER CAUSED AND REGARDLESS\nOF THE THEORY OF LIABILITY, ARISING OUT OF OR IN CONNECTION\nWITH THE USE OR PERFORMANCE OF THIS SOFTWARE.\n\n\nPyWin32 (win32dlgdyn)\n---------------------\n\nCopyright (C) 1995 by Motek Information Systems, Beverly Hills, CA, USA\n\n                      All Rights Reserved\n\nPermission to use, copy, modify, and distribute this software and its \ndocumentation for any purpose and without fee is hereby granted, \nprovided that the above copyright notice and the two paragraphs following\nit appear in all copies, and that the name of Motek Information Systems\nnot be used in advertising or publicity pertaining to distribution of the\nsoftware without specific, written prior permission.\n\nMOTEK INFORMATION SYSTEMS DISCLAIMS ALL WARRANTIES WITH REGARD TO\nTHIS SOFTWARE, INCLUDING ALL IMPLIED WARRANTIES OF MERCHANTABILITY AND\nFITNESS, IN NO EVENT SHALL MOTEK BE LIABLE FOR ANY SPECIAL, INDIRECT OR\nCONSEQUENTIAL DAMAGES OR ANY DAMAGES WHATSOEVER RESULTING FROM LOSS OF USE,\nDATA OR PROFITS, WHETHER IN AN ACTION OF CONTRACT, NEGLIGENCE OR OTHER\nTORTIOUS ACTION, ARISING OUT OF OR IN CONNECTION WITH THE USE OR\nPERFORMANCE OF THIS SOFTWARE.\n\n\nPyWin32 (stdin)\n---------------\n\nCopyright (c) 2000 David Abrahams. Permission to copy, use, modify, sell\nand distribute this software is granted provided this copyright\nnotice appears in all copies. This software is provided \"as is\" without\nexpress or implied warranty, and with no claim as to its suitability for\nany purpose.\n\n\nPillow\n------\n\nThe Python Imaging Library (PIL) is\n\n   Copyright (c) 1997-2011 by Secret Labs AB \n   Copyright (c) 1995-2011 by Fredrik Lundh\n\nBy obtaining, using, and/or copying this software and/or its associated\ndocumentation, you agree that you have read, understood, and will comply\nwith the following terms and conditions:\n\nPermission to use, copy, modify, and distribute this software and its\nassociated documentation for any purpose and without fee is hereby\ngranted, provided that the above copyright notice appears in all copies,\nand that both that copyright notice and this permission notice appear in\nsupporting documentation, and that the name of Secret Labs AB or the\nauthor not be used in advertising or publicity pertaining to\ndistribution of the software without specific, written prior permission.\n\nSECRET LABS AB AND THE AUTHOR DISCLAIMS ALL WARRANTIES WITH REGARD TO\nTHIS SOFTWARE, INCLUDING ALL IMPLIED WARRANTIES OF MERCHANTABILITY AND\nFITNESS. IN NO EVENT SHALL SECRET LABS AB OR THE AUTHOR BE LIABLE FOR\nANY SPECIAL, INDIRECT OR CONSEQUENTIAL DAMAGES OR ANY DAMAGES WHATSOEVER\nRESULTING FROM LOSS OF USE, DATA OR PROFITS, WHETHER IN AN ACTION OF\nCONTRACT, NEGLIGENCE OR OTHER TORTIOUS ACTION, ARISING OUT OF OR IN\nCONNECTION WITH THE USE OR PERFORMANCE OF THIS SOFTWARE.\n\n\nPillow (QuantOctree)\n--------------------\n\nCopyright (c) 2010 Oliver Tonnhofer <olt@bogosoft.com>, Omniscale\n\nPermission is hereby granted, free of charge, to any person obtaining a copy\nof this software and associated documentation files (the \"Software\"), to deal\nin the Software without restriction, including without limitation the rights\nto use, copy, modify, merge, publish, distribute, sublicense, and/or sell\ncopies of the Software, and to permit persons to whom the Software is\nfurnished to do so, subject to the following conditions:\n\nThe above copyright notice and this permission notice shall be included in\nall copies or substantial portions of the Software.\n\nTHE SOFTWARE IS PROVIDED \"AS IS\", WITHOUT WARRANTY OF ANY KIND, EXPRESS OR\nIMPLIED, INCLUDING BUT NOT LIMITED TO THE WARRANTIES OF MERCHANTABILITY,\nFITNESS FOR A PARTICULAR PURPOSE AND NONINFRINGEMENT. IN NO EVENT SHALL THE\nAUTHORS OR COPYRIGHT HOLDERS BE LIABLE FOR ANY CLAIM, DAMAGES OR OTHER\nLIABILITY, WHETHER IN AN ACTION OF CONTRACT, TORT OR OTHERWISE, ARISING FROM,\nOUT OF OR IN CONNECTION WITH THE SOFTWARE OR THE USE OR OTHER DEALINGS IN\nTHE SOFTWARE.\n\n\nPsUtil\n------\n\nCopyright (c) 2009, Jay Loden, Dave Daeschler, Giampaolo Rodola'\nAll rights reserved.\n\nRedistribution and use in source and binary forms, with or without modification,\nare permitted provided that the following conditions are met:\n\nRedistributions of source code must retain the above copyright notice, this\n   list of conditions and the following disclaimer.\nRedistributions in binary form must reproduce the above copyright notice,\n   this list of conditions and the following disclaimer in the documentation\n   and/or other materials provided with the distribution.\nNeither the name of the psutil authors nor the names of its contributors\n   may be used to endorse or promote products derived from this software without\n   specific prior written permission.\n\nTHIS SOFTWARE IS PROVIDED BY THE COPYRIGHT HOLDERS AND CONTRIBUTORS \"AS IS\" AND\nANY EXPRESS OR IMPLIED WARRANTIES, INCLUDING, BUT NOT LIMITED TO, THE IMPLIED\nWARRANTIES OF MERCHANTABILITY AND FITNESS FOR A PARTICULAR PURPOSE ARE\nDISCLAIMED. IN NO EVENT SHALL THE COPYRIGHT OWNER OR CONTRIBUTORS BE LIABLE FOR\nANY DIRECT, INDIRECT, INCIDENTAL, SPECIAL, EXEMPLARY, OR CONSEQUENTIAL DAMAGES\n(INCLUDING, BUT NOT LIMITED TO, PROCUREMENT OF SUBSTITUTE GOODS OR SERVICES;\nLOSS OF USE, DATA, OR PROFITS; OR BUSINESS INTERRUPTION) HOWEVER CAUSED AND ON\nANY THEORY OF LIABILITY, WHETHER IN CONTRACT, STRICT LIABILITY, OR TORT\n(INCLUDING NEGLIGENCE OR OTHERWISE) ARISING IN ANY WAY OUT OF THE USE OF THIS\nSOFTWARE, EVEN IF ADVISED OF THE POSSIBILITY OF SUCH DAMAGE.\n\n\nPython-Dateutil\n---------------\n\nCopyright (c) 2003-2011 - Gustavo Niemeyer <gustavo@niemeyer.net>\nCopyright (c) 2012-2014 - Tomi Pieviläinen <tomi.pievilainen@iki.fi>\nCopyright (c) 2014      - Yaron de Leeuw <me@jarondl.net>\n\nAll rights reserved.\n\nRedistribution and use in source and binary forms, with or without\nmodification, are permitted provided that the following conditions are met:\n\n   Redistributions of source code must retain the above copyright notice,\n      this list of conditions and the following disclaimer.\n   Redistributions in binary form must reproduce the above copyright notice,\n      this list of conditions and the following disclaimer in the documentation\n      and/or other materials provided with the distribution.\n   Neither the name of the copyright holder nor the names of its\n      contributors may be used to endorse or promote products derived from\n      this software without specific prior written permission.\n\nTHIS SOFTWARE IS PROVIDED BY THE COPYRIGHT HOLDERS AND CONTRIBUTORS\n\"AS IS\" AND ANY EXPRESS OR IMPLIED WARRANTIES, INCLUDING, BUT NOT\nLIMITED TO, THE IMPLIED WARRANTIES OF MERCHANTABILITY AND FITNESS FOR\nA PARTICULAR PURPOSE ARE DISCLAIMED. IN NO EVENT SHALL THE COPYRIGHT OWNER OR\nCONTRIBUTORS BE LIABLE FOR ANY DIRECT, INDIRECT, INCIDENTAL, SPECIAL,\nEXEMPLARY, OR CONSEQUENTIAL DAMAGES (INCLUDING, BUT NOT LIMITED TO,\nPROCUREMENT OF SUBSTITUTE GOODS OR SERVICES; LOSS OF USE, DATA, OR\nPROFITS; OR BUSINESS INTERRUPTION) HOWEVER CAUSED AND ON ANY THEORY OF\nLIABILITY, WHETHER IN CONTRACT, STRICT LIABILITY, OR TORT (INCLUDING\nNEGLIGENCE OR OTHERWISE) ARISING IN ANY WAY OUT OF THE USE OF THIS\nSOFTWARE, EVEN IF ADVISED OF THE POSSIBILITY OF SUCH DAMAGE.\n\n\nPython-Six\n----------\n\nCopyright (c) 2010-2014 Benjamin Peterson\n\nPermission is hereby granted, free of charge, to any person obtaining a copy of\nthis software and associated documentation files (the \"Software\"), to deal in\nthe Software without restriction, including without limitation the rights to\nuse, copy, modify, merge, publish, distribute, sublicense, and/or sell copies of\nthe Software, and to permit persons to whom the Software is furnished to do so,\nsubject to the following conditions:\n\nThe above copyright notice and this permission notice shall be included in all\ncopies or substantial portions of the Software.\n\nTHE SOFTWARE IS PROVIDED \"AS IS\", WITHOUT WARRANTY OF ANY KIND, EXPRESS OR\nIMPLIED, INCLUDING BUT NOT LIMITED TO THE WARRANTIES OF MERCHANTABILITY, FITNESS\nFOR A PARTICULAR PURPOSE AND NONINFRINGEMENT. IN NO EVENT SHALL THE AUTHORS OR\nCOPYRIGHT HOLDERS BE LIABLE FOR ANY CLAIM, DAMAGES OR OTHER LIABILITY, WHETHER\nIN AN ACTION OF CONTRACT, TORT OR OTHERWISE, ARISING FROM, OUT OF OR IN\nCONNECTION WITH THE SOFTWARE OR THE USE OR OTHER DEALINGS IN THE SOFTWARE.\n\n\n"
  # "About"
  # "The Advanced Plotting Toolkit was developed by Heliosphere Research LLC, a small consulting and software development company located in Boulder Colorado.\n\nCopyright (c) 2014-2015 Heliosphere Research LLC.\n\n\nWe gratefully acknowledge the use of the Matplotlib 2D plotting library. An embedded version of Matplotlib is the foundation of the plotting system used in the Toolkit.  Heliosphere is proud to participate in the Matplotlib ecosystem, which is made up of thousands of scientists, engineers and developers across the world."
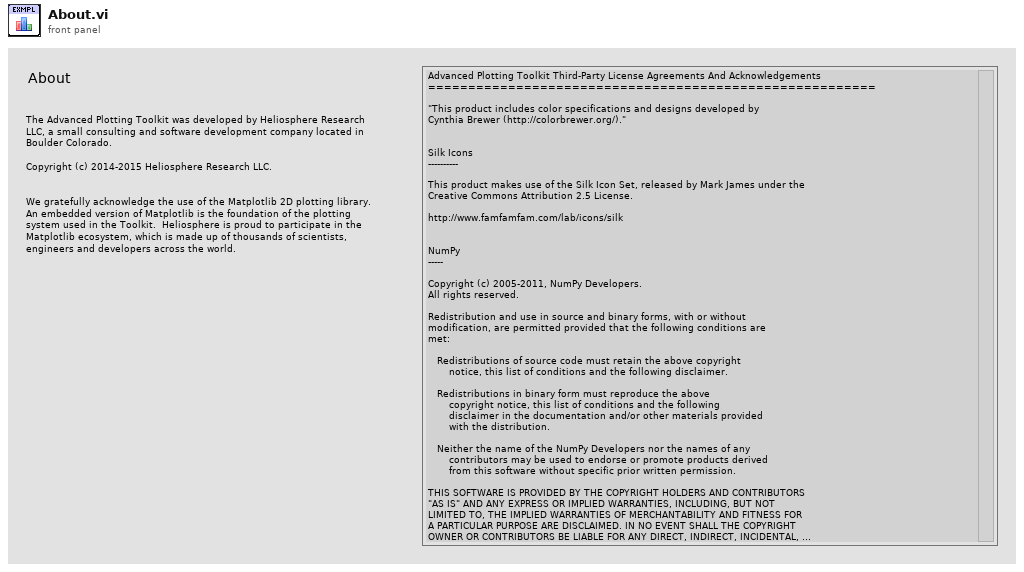
[diagram p1: front panel]
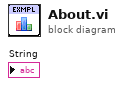
[diagram p0: block diagram]
diagram:
